vi "4Ch Interleaved Fxp to wfms.vi"(0 "reference in":refnum<class "Fcurve.lvclass">, 2 "Wfms (4in)":fxp<+/-,27,5>[](array[numeric]), 5 "error in (no error)":errorcluster) -> (14 "reference out":refnum<class "Fcurve.lvclass">, 16 "Wfms (4out)":waveform(dbl)[](array[waveform]), 19 "error out":errorcluster)   [LabVIEW 2019, in "Fcurve.lvclass"]
doc: "Gets the raw data of index 0 and 1 of the interleaved waveform channel and outputs it as an array for 2 channels"
uses:
  Fcurve.lvclass
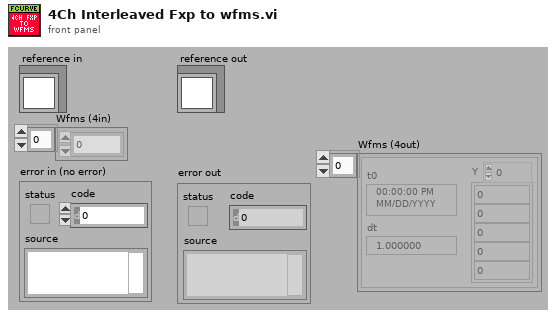
[diagram p1: front panel]
types:
  T1 = typedef "Fcurve.lvclass/ObjectAttributes.ctl" = cluster{"MyAttribute":dbl, "Fcurve Metadata":T2, "Contact Spread of dev":dbl, "Tau Delay (ms)":dbl, "Points of contact":dbl, "Def_wfm":cluster{"Max":dbl, "Min":dbl}, "Zpos_wfm":cluster{"Max":dbl, "Min":dbl}, "Contact stat?":bool, "Real AI dt (s)":dbl, "Decimation":cluster{"App":cluster{"Dec":i32, "apply":bool}, "Con":cluster{"Dec":i32, "apply":bool}, "Ret":cluster{"Dec":i32, "apply":bool}}, "Segment def[0]":dbl, "Segment Zpos[0]":dbl, "Raw Datum":waveform(dbl)[], "Group metadata":T3, "M_data obj":refnum<class "metadata.lvclass">, "Channel name(s)":string[], "Segment fcurve data":cluster{"X":dbl[], "Y":dbl[]}[], "Segment duration":cluster{"Start":i32, "Duration":i32}[], "Segment info":T4[], "Segment durations (S)":dbl[], "Segments Maxmin":T6[]}
  T2 = typedef "Fcurve.lvclass/Metadata.ctl" = cluster{"dt (us)":dbl, "Dec Factor":dbl, "Z piezo Sensitivity (nm/V)":dbl, "K (N/m)":dbl, "Sp (V)":dbl, "Contact (ms)":dbl, "Zpos contact":dbl, "Vel_app (nm/s)":dbl, "Vel_ret (nm/s)":dbl, "deltaV (nm)":dbl, "Def_V0 (v)":dbl, "Piezo gain":dbl, "invOLS (nm/V)":dbl}
  T3 = typedef "TDMS_DataHandler.lvclass/Fcurve Meta data.ctl" = cluster{"property names":string[], "property values":variant[]}
  T4 = typedef "Fcurve.lvclass/Fcurve segments --cluster.ctl" = cluster{"type":T5, "nb points":i32, "dec factor":u32, "sampling rate (S/s)":u32}
  T5 = typedef "metadata.lvclass/Segment type--combobox.ctl" = string
  T6 = typedef "Fcurve.lvclass/Segment MaxMin --cluster.ctl" = cluster{"Def":cluster{"max value":dbl, "min value":dbl}, "Zpos":cluster{"max value":dbl, "min value":dbl}}
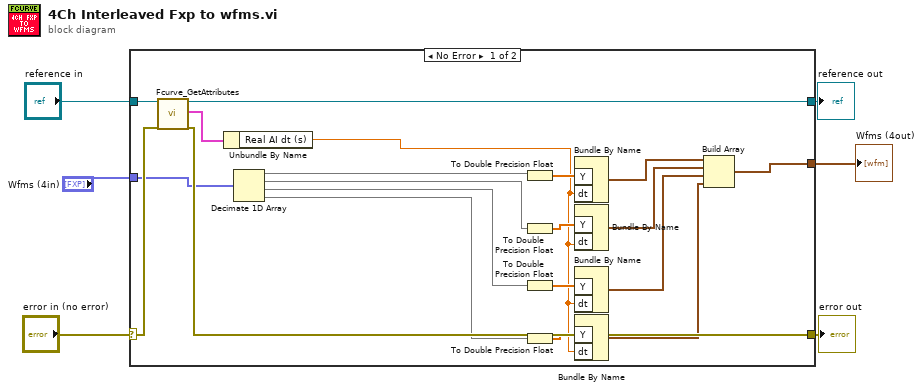
[diagram p0: block diagram]
diagram:
  n1 = case shown="No Error" "error in (no error)" {
    selector: "error in (no error)" -> [w24 w28]
    tunnel: [w23 w28] -> w5
    tunnel: [w25 w27] -> w3
    tunnel: "reference in" -> [w26 w27]
    tunnel: "Wfms (4in)" -> [w17 _]
    tunnel: [w15 _] -> w1
    frame No Error {
      n2 = call "Fcurve_GetAttributes.vi"("reference in"=w26, "error in (no error)"=w24) -> ("reference out"=w25:refnum<class "Fcurve.lvclass">, "attributes"=w22:T1, "error out"=w23:errorcluster)  [unwired: 14 in, 1 out]
      n3 = Unbundle By Name(w22) -> ("Real AI dt (s)"=w9:dbl)
      n4 = Decimate 1D Array(w17) -> (w20:fxp<+/-,27,5>[], w21:fxp<+/-,27,5>[], w11:fxp<+/-,27,5>[], w10:fxp<+/-,27,5>[])
      n5 = To Double Precision Float(number=w20) -> (double precision float=w19:dbl[])
      n6 = To Double Precision Float(number=w21) -> (double precision float=w18:dbl[])
      n7 = To Double Precision Float(number=w11) -> (double precision float=w13:dbl[])
      n8 = To Double Precision Float(number=w10) -> (double precision float=w14:dbl[])
      n9 = Bundle By Name("Y"=w19, "dt"=w9) -> (w16:waveform(dbl))  [unwired: 1 in]
      n10 = Bundle By Name("Y"=w18, "dt"=w9) -> (w12:waveform(dbl))  [unwired: 1 in]
      n11 = Bundle By Name("Y"=w13, "dt"=w9) -> (w8:waveform(dbl))  [unwired: 1 in]
      n12 = Bundle By Name("Y"=w14, "dt"=w9) -> (w7:waveform(dbl))  [unwired: 1 in]
      n13 = Build Array(w16, w12, w8, w7) -> (w15:waveform(dbl)[])
    }
    frame Error {
    }
  }
  "error out" <- w5
  "reference out" <- w3
  "Wfms (4out)" <- w1
